vi "Find_Beam_Max_Pos.vi"(3 "Mode":T5, 4 "Beams to peak up":i32[](array[numeric]), 5 "Traverse line In":T2 {"Carrier_2 Q (l/min)" format="%#.2f"; "Row Duration (mins)" format="%#.1f"; "Row No" min=0; "Trace Gas Concentration (%)" min=0.0 format="%#_4f"; "Carrier_1 Q (l/min)" format="%#.4f"; "Start X" format="%#.2f"; "Start Y" format="%#.2f"; "Start Z" format="%#.2f"; "End X" format="%#.2f"; "End Y" format="%#.2f"; "End Z" format="%#.2f"; "Tunnel Speed" format="%#.2f"; "Averaging time (mins)" min=0.0 format="%#.2f"}) -> (0 "Error Message":string, 1 "Status":T1, 2 "Traverse line Out":T2 {"Carrier_2 Q (l/min)" format="%#.2f"; "Row Duration (mins)" format="%#.1f"; "Row No" min=0; "Trace Gas Concentration (%)" min=0.0 format="%#_4f"; "Carrier_1 Q (l/min)" format="%#.4f"; "Start X" format="%#.2f"; "Start Y" format="%#.2f"; "Start Z" format="%#.2f"; "End X" format="%#.2f"; "End Y" format="%#.2f"; "End Z" format="%#.2f"; "Tunnel Speed" format="%#.2f"; "Averaging time (mins)" min=0.0 format="%#.2f"})   [LabVIEW 2020]
uses:
  Gen Trav/Traverse_cluster.ctl
  Gen Trav/Spacing.ctl
  Controls/Multi_run_mode.ctl
  Controls/User_Specific_mode.ctl
  Gen Trav/Multi_Run_Status.ctl
  ADAM Client/Sub VIs/ADAM Controls/Remember_value_mode.ctl
  Gen Trav/Trav_mode.ctl
  Controls/Tunnel_Coordinates.ctl
  Globals/Meas_global.vi
  Globals/Preference_global.vi
  Utilities/Email_transfer_global.vi
panel:
  out "Beam Number":i32
  out "Traverse Name":string
  out "Picture Log":path
  out "First Call":bool
  out "Beam Data":dbl[][](array[numeric]) format="%.2f"
  in  "Index":i32
  # "X                Y                 Z        Datum Power"
  # "Green Unshifted\nGreen Shifted\nBlue Unshifted\nBlue Shifted"
  # "X           Y          Z"
  # "Start"
  # "End"
  # "X           Y          Z"
  # "Start"
  # "End"
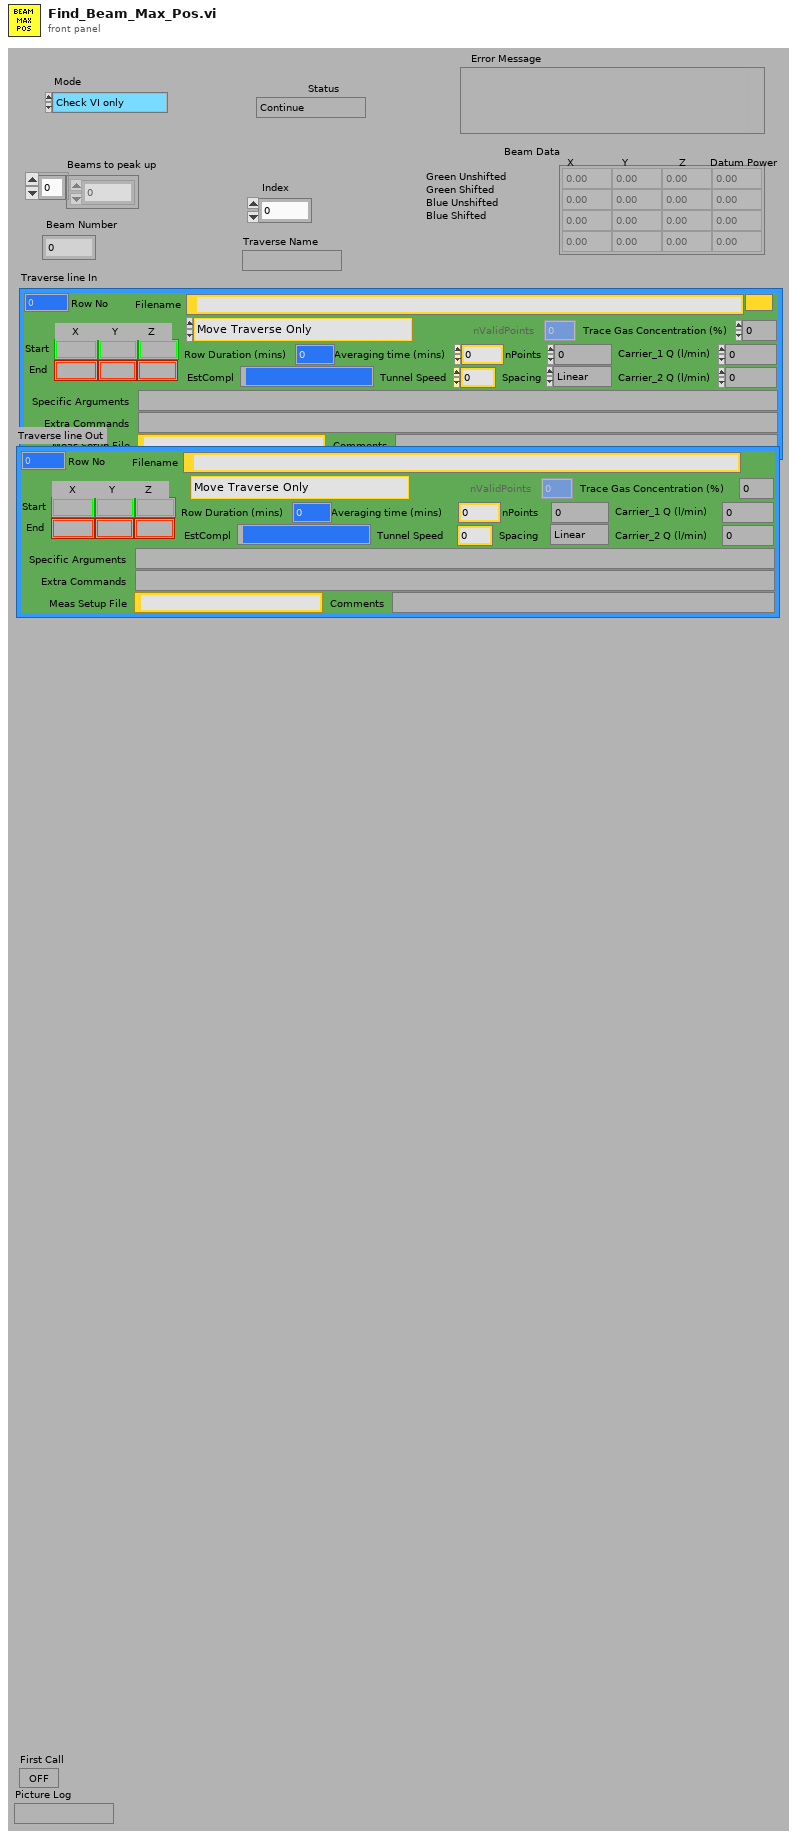
[diagram p1: front panel]
types:
  T1 = typedef "Multi_Run_Status.ctl" = enum16{"Continue", "Continue with Error", "Jump to Next Point", "Jump to Next Row", "Jump To Fall Back", "Terminate Run"}
  T2 = typedef "Traverse_cluster.ctl" = cluster{"Start X":sgl, "Start Y":sgl, "Start Z":sgl, "End X":sgl, "End Y":sgl, "End Z":sgl, "nPoints":i32, "Spacing":T3, "Filename":path, "Tunnel Speed":dbl, "Averaging time (mins)":dbl, "Extra Commands":string, "Carrier_1 Q (l/min)":dbl, "Carrier_2 Q (l/min)":dbl, "Trace Gas Concentration (%)":dbl, "Specific Arguments":string, "Comments":string, "Row No":i32, "Row Type Selector":T4, "EstCompl":string, "Row Duration (mins)":dbl, "nValidPoints":i32, "Meas Setup File":string}
  T3 = typedef "Spacing.ctl" = enum16{"Linear", "Log", "Gauss", "Specified", "N/A"}
  T4 = typedef "Multi_run_mode.ctl" = enum16{"Move Traverse Only", "Set Tunnel Speed Only", "Set Source Only", "Set Measurement Conditions", "Single Measurement", "Vertical Profile", "Lateral Profile", "Longitudinal Profile", "Multi-Axis Profile", "Explore Volume", "Auto Calibrate", "Meas Fast FID Bkgnd", "Check Beam Power", "Scanning Valve Measurement", "Run VI Named:", "Set ADAM Ch", "Wait (minutes)", "Send Message", "Synchronize With:", "Fall Back to this Row", "Turn Off Row Repeating", "Traverse 3D Volume", "Blank Row", "Jump to Fall Back Row"}
  T5 = typedef "User_Specific_mode.ctl" = enum16{"Check VI only", "Run VI"}
  T6 = typedef "Fixed Axis.ctl" = enum16{"X Axis Fixed", "Y Axis Fixed", "Z Axis Fixed"}
  T7 = cluster{"Position":dbl[], "Traverse Name":string}[][]
  T8 = typedef "Remember_value_mode.ctl" = enum16{"Read only", "Read and Write"}
  T9 = typedef "Tunnel_Coordinates.ctl" = enum16{"Work in Tunnel Coordinates", "Work in Model Coordinates"}
  T10 = typedef "Trav_mode.ctl" = enum16{"Move traverse", "Read traverse position", "Teach Position"}
  T11 = cluster{"second":i32, "minute":i32, "hour":i32, "day of month":i32, "month":i32, "year":i32, "day of week":i32, "day of year":i32, "is DST":i32}
  T12 = cluster{"Position":dbl[], "Traverse Name":string}[]
  T13 = cluster{"Position":dbl[], "Traverse Name":string}
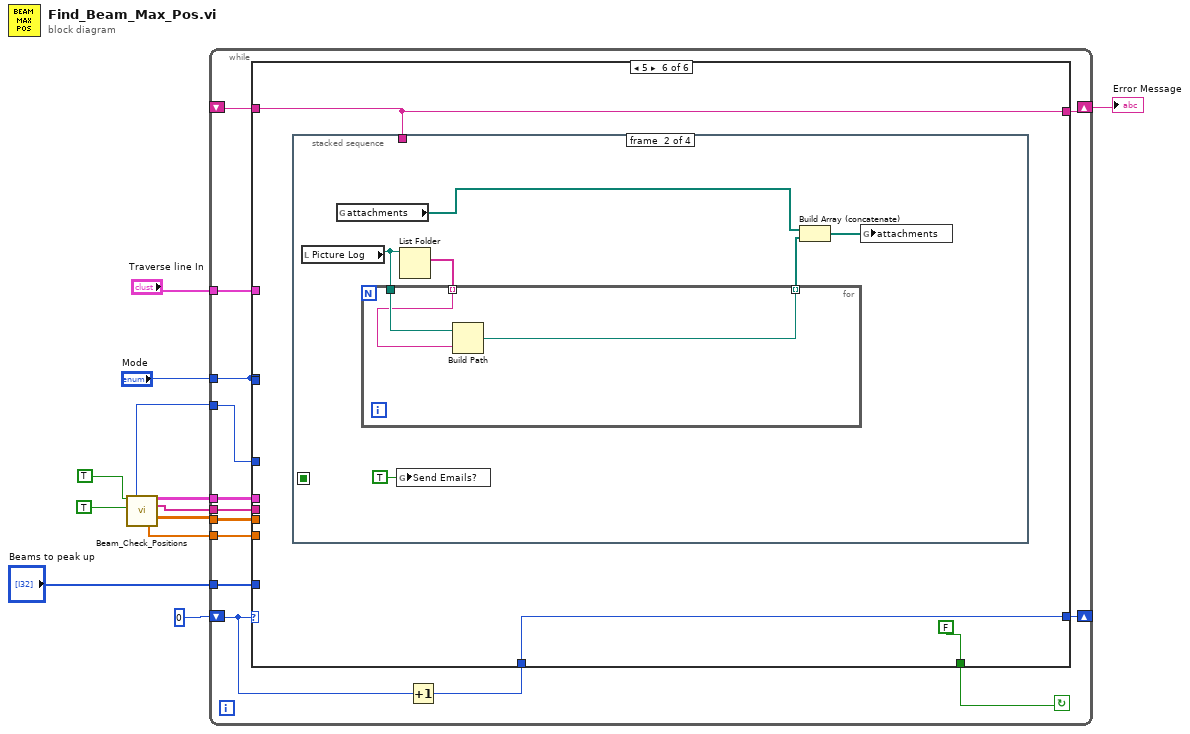
[diagram p0: block diagram]
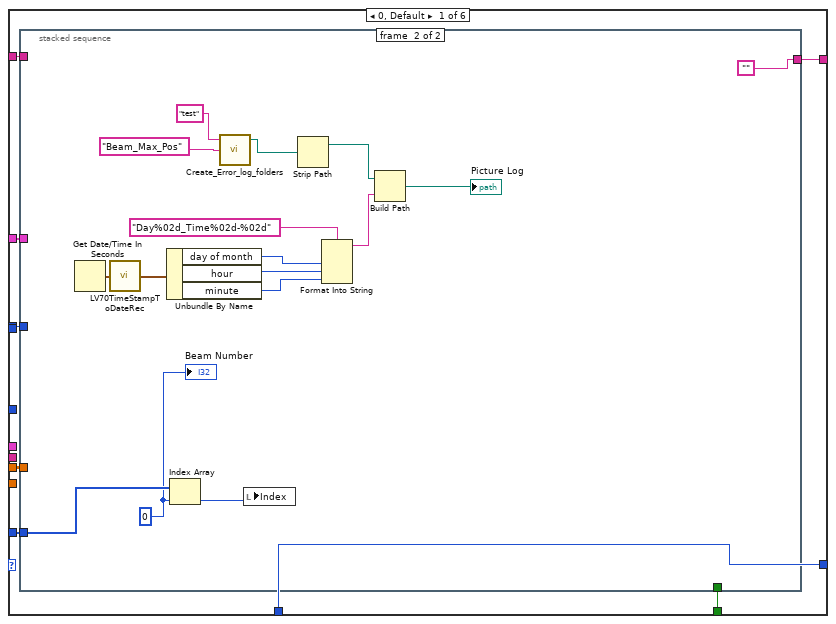
[diagram p2: hidden frame]
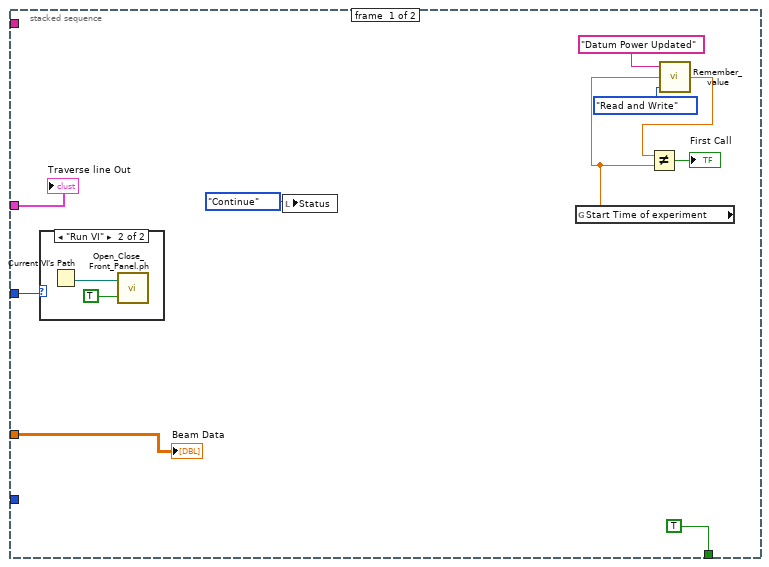
[diagram p3: hidden frame]
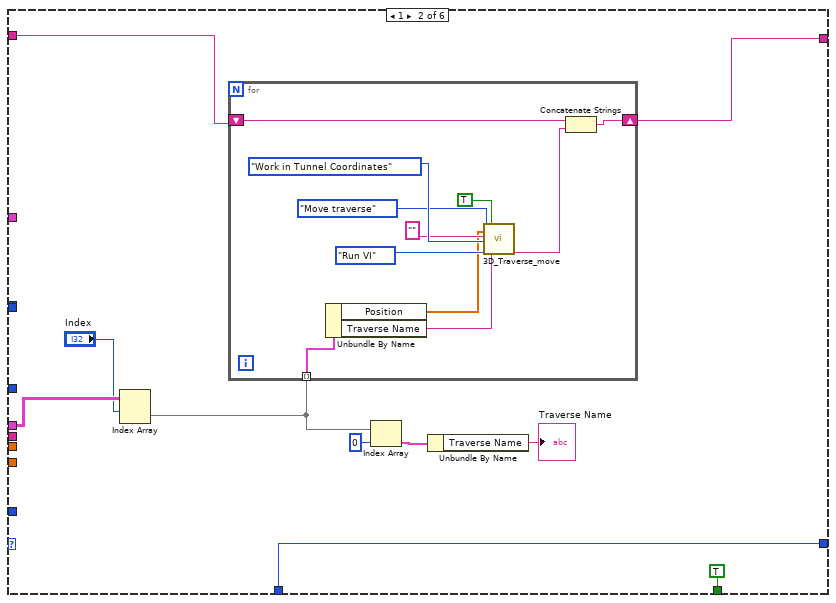
[diagram p5: hidden frame]
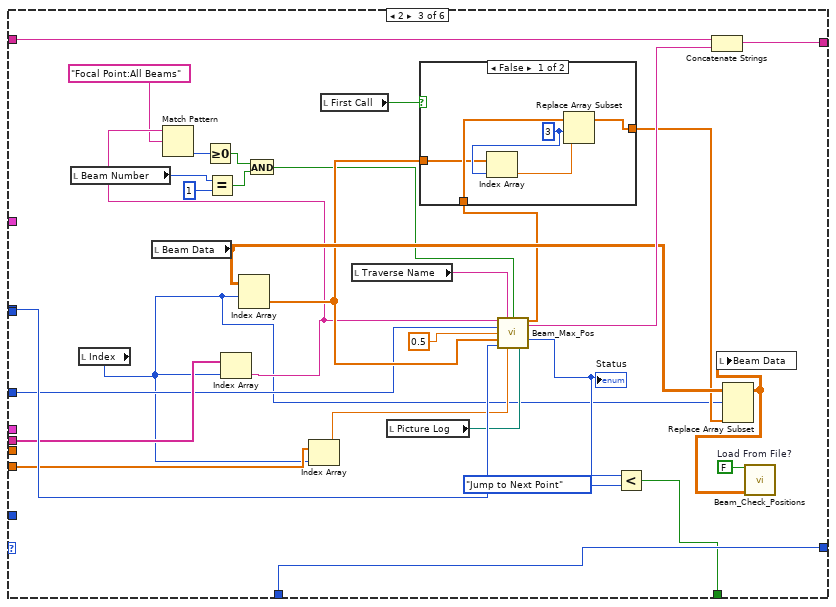
[diagram p6: hidden frame]
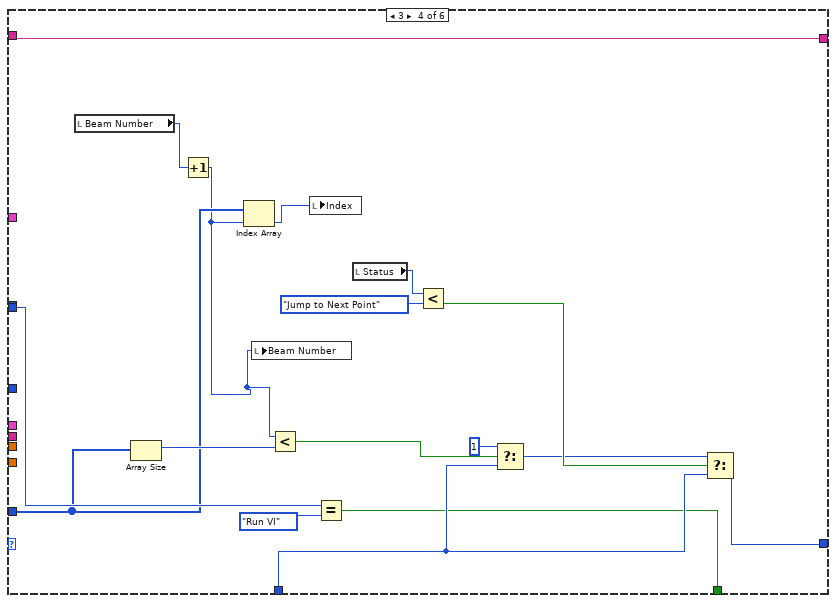
[diagram p8: hidden frame]
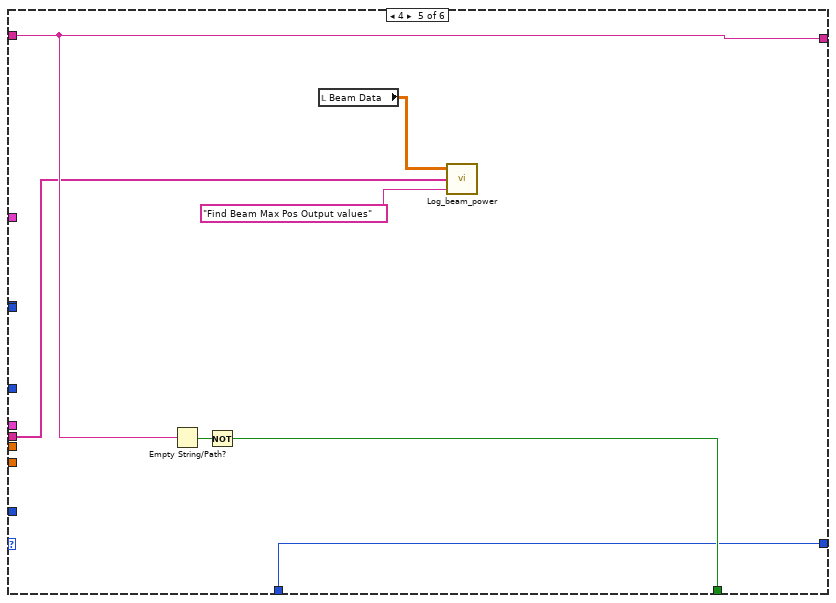
[diagram p9: hidden frame]
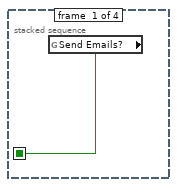
[diagram p10: hidden frame]
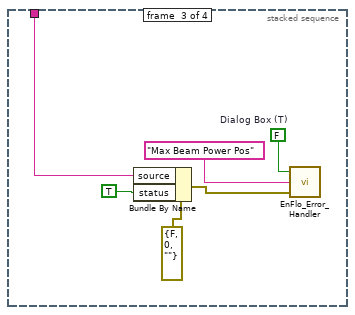
[diagram p11: hidden frame]
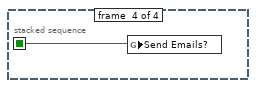
[diagram p12: hidden frame]
diagram:
  n1 = call "Beam_Check_Positions.vi"("Load From File?"=TRUE, "Give Focal Point Info (F)"=TRUE) -> ("Fixed Axis"=w8:T6, "Beam Info"=w5:T7, "Beam Names"=w2:string[], "Primary Beam Positions"=w4:dbl[][], "Wavelength (nm)"=w3:dbl[])  [unwired: 5 in, 4 out]
  n2 = while {
    shift-left: _ -> [w19]
    shift-right: [w20] -> w7
    tunnel: "Traverse line In" -> [w25]
    tunnel: "Mode" -> [w21]
    shift-left: 0 -> [w26]
    shift-right: [w22] -> _
    tunnel: w2 -> [w18]
    tunnel: w3 -> [w17]
    tunnel: w4 -> [w16]
    tunnel: w5 -> [w15]
    tunnel: w8 -> [w14]
    tunnel: "Beams to peak up" -> [w13]
    stop <- w24 continue-if-true
    n3 = Increment(x=w26) -> (x+1=w23:i32)
    n4 = case shown="5" w26 {
      tunnel: w25 -> [w31 _ _ _ _ _]
      tunnel: w21 -> [w33 _ w113 _ _ _]
      tunnel: [w32 TRUE w107 w129 w140 FALSE] -> w24
      tunnel: w23 -> [w34 w64 w114 w133 w139 w147]
      tunnel: [w34 w64 w114 w132 w139 w147] -> w22
      tunnel: w21 -> [_ _ _ w130 _ _]
      tunnel: [w30 w65 w110 w127 w142 w145] -> w20
      tunnel: w19 -> [w28 w66 w112 w127 w142 w145]
      tunnel: w18 -> [_ _ w98 _ w138 _]
      tunnel: w17 -> [_ _ w97 _ _ _]
      tunnel: w16 -> [w29 _ _ _ _ _]
      tunnel: w15 -> [_ w68 _ _ _ _]
      tunnel: w14 -> [_ _ w94 _ _ _]
      tunnel: w13 -> [w27 _ _ w123 _ _]
      frame 0, Default {
        n5 = stacked-sequence {
          tunnel: w33 -> [w43 _]
          tunnel: [TRUE _] -> w32
          tunnel: w31 -> [w42 _]
          tunnel: [_ ""] -> w30
          tunnel: w29 -> [w36 _]
          tunnel: w28 -> [_ _]
          tunnel: w27 -> [_ w49]
          frame #0 {
            n6 = case shown="\"Run VI\"" w43 {
              frame "Check VI only" {
              }
              frame "Run VI" {
                n7 = Current VI's Path() -> (path=w45:path)
                n8 = call "Open_Close_Front_Panel.ph.vi"("openWindow (T)"=TRUE ("Front Panel Window:Open"), "VI path"=w45) -> ()  [unwired: 2 out]
              }
            }
            n9 = local write "Status"(Multi_Run_Status."Continue" ("Status")) -> ()
            n10 = global read "Meas_global.vi" "Start Time of experiment"() -> (w38:dbl)
            n11 = call "Remember_value.vi"("Mode"=Remember_value_mode."Read and Write", "Input Value"=w38, "Ch name"="Datum Power Updated") -> ("Output Value"=w39:dbl)
            n12 = Not Equal?(x=w39, y=w38) -> (x != y?=→"First Call":bool)
            "Beam Data" <- w36
            "Traverse line Out" <- w42
          }
          frame #1 {
            w47 = 0 ("Index")
            n13 = Get Date/Time In Seconds() -> (seconds since 1Jan1904=w52:timestamp)
            n14 = call <vilib>:"LV70TimeStampToDateRec.vi"("time stamp"=w52) -> ("date time rec"=w60:T11)
            n15 = Unbundle By Name(w60) -> ("day of month"=w57:i32, "hour"=w58:i32, "minute"=w59:i32)
            n16 = Index Array(array=w49, index=w47) -> (element=w48:i32)
            n17 = call "Create_Error_log_folders.vi"("Log Filename"="test", "Log Folder"="Beam_Max_Pos" ("name or relative path")) -> ("Local Log File"=w51:path)  [unwired: 4 in, 1 out]
            n18 = local write "Index"(w48) -> ()
            n19 = Strip Path(path=w51) -> (stripped path=w61:path)  [unwired: 1 out]
            n20 = Format Into String(format string="Day%02d_Time%02d-%02d", w57, w58, w59) -> (resulting string=w62:string)  [unwired: 2 in, 1 out]
            n21 = Build Path(base path=w61, name or relative path=w62) -> (appended path=→"Picture Log":path)
            "Beam Number" <- w47
          }
        }
      }
      frame 1 {
        n22 = Index Array(array=w68, index (row)="Index") -> (element=w72:T12)  [unwired: 1 in]
        n23 = for {
          tunnel: w72 -> [w78] mode=indexing
          shift-right: [w75] -> w65
          shift-left: w66 -> [w74]
          n24 = Unbundle By Name(w78) -> ("Position"=w77:dbl[], "Traverse Name"=w76:string)
          n25 = call "3D_Traverse_move.vi"("Mode"=Trav_mode."Move traverse", "Position"=w77, "Extra command String"="", "Work in Tunnel Coordinates"=Tunnel_Coordinates."Work in Tunnel Coordinates", "Simulate/Run"=User_Specific_mode."Run VI", "Route Checking?"=TRUE, "Traverse name"=w76) -> ("Error String"=w73:string)  [unwired: 9 in, 3 out]
          n26 = Concatenate Strings(w74, w73) -> (w75:string)
        }
        n27 = Index Array(array=w72, index=0) -> (element=w71:T13)
        n28 = Unbundle By Name(w71) -> ("Traverse Name"=→"Traverse Name":string)
      }
      frame 2 {
        w99 = FALSE  # Load From File?
        n29 = local read "Beam Number"() -> (w87:i32)
        n30 = local read "Index"() -> (w89:i32)
        n31 = local read "Beam Data"() -> (w105:dbl[][])
        n32 = Equal?(x=w87, y=1) -> (x = y?=w85:bool)
        n33 = Index Array(array=w98, index=w89) -> (element=w92:string)
        n34 = Match Pattern(string=w92, regular expression="Focal Point:All Beams") -> (offset past match=w90:i32)  [unwired: 1 in, 3 out]
        n35 = Greater Or Equal To 0?(x=w90) -> (x >= 0?=w86:bool)
        n36 = Index Array(array=w105, index (row)=w89) -> (element=w100:dbl[])  [unwired: 1 in]
        n37 = And(x=w86, y=w85) -> (x .and. y?=w84:bool)
        n38 = Index Array(array=w97, index=w89) -> (element=w96:dbl)
        n39 = local read "First Call"() -> (w104:bool)
        n40 = local read "Traverse Name"() -> (w95:string)
        n41 = local read "Picture Log"() -> (w106:path)
        n42 = call "Beam_Max_Pos.vi"("Beam Name"=w92, "Traverse Name"=w95, "Fixed Axis only?"=w84, "Fixed Axis"=w94, "Search Step (mm)"=0.5, "Starting Position"=w100, "Mode"=w113, "Wavelength  nm"=w96, "Picture Log"=w106) -> ("Message"=w111:string, "Beam maxima"=w102:dbl[], "Status"=w108:T1)  [unwired: 3 in, 1 out]
        "Status" <- w108
        n43 = case shown="False" w104 {
          tunnel: [w118 w120] -> w103
          tunnel: w102 -> [w119 w120]
          tunnel: w100 -> [w116 _]
          frame False {
            w117 = 3 ("index")
            n44 = Index Array(array=w116, index=w117) -> (element=w115:dbl)
            n45 = Replace Array Subset(array=w119, new element=w115, index=w117) -> (w118:dbl[])
          }
          frame True {
          }
        }
        n46 = Less?(x=w108, y=Multi_Run_Status."Jump to Next Point" ("Status")) -> (x < y?=w107:bool)
        n47 = Concatenate Strings(w112, w111) -> (w110:string)
        n48 = Replace Array Subset(array=w105, new element=w103, index (row)=w89) -> (w101:dbl[][])  [unwired: 1 in]
        n49 = local write "Beam Data"(w101) -> ()
        n50 = call "Beam_Check_Positions.vi"("Load From File?"=w99, "Primary Positions In"=w101) -> ()  [unwired: 5 in, 9 out]
      }
      frame 3 {
        n51 = local read "Beam Number"() -> (w124:i32)
        n52 = Array Size(array=w123) -> (size(s)=w126:i32)
        n53 = Increment(x=w124) -> (x+1=w122:i32)
        n54 = Index Array(array=w123, index=w122) -> (element=w121:i32)
        n55 = local write "Beam Number"(w122) -> ()
        n56 = Less?(x=w122, y=w126) -> (x < y?=w125:bool)
        n57 = local write "Index"(w121) -> ()
        n58 = Equal?(x=w130, y=User_Specific_mode."Run VI" ("Mode")) -> (x = y?=w129:bool)
        n59 = local read "Status"() -> (w137:T1)
        n60 = Less?(x=w137, y=Multi_Run_Status."Jump to Next Point" ("Status")) -> (x < y?=w135:bool)
        n61 = Select(t=1, s=w125, f=w133) -> (s? t:f=w134:i32)
        n62 = Select(t=w134, s=w135, f=w133) -> (s? t:f=w132:i32)
      }
      frame 4 {
        n63 = Empty String/Path?(string/path=w142) -> (empty?=w141:bool)
        n64 = Not(x=w141) -> (.not. x?=w140:bool)
        n65 = local read "Beam Data"() -> (w144:dbl[][])
        n66 = call "Log_beam_power.vi"("Message"="Find Beam Max Pos Output values", "Beam Names"=w138, "Beam Data"=w144) -> ()  [unwired: 3 out]
      }
      frame 5 {
        n67 = stacked-sequence {
          seq-local: [w148 _ _ _] -> [_ _ _ w164]
          tunnel: w145 -> [_ _ w158 _]
          frame #0 {
            n68 = global read "Preference_global.vi" "Send Emails?"() -> (w148:bool)
          }
          frame #1 {
            n69 = local read "Picture Log"() -> (w151:path)
            n70 = global read "Email_transfer_global.vi" "attachments"() -> (w152:path[])
            n71 = global write "Preference_global.vi" "Send Emails?"(TRUE ("Send Emails?")) -> ()
            n72 = List Folder(path=w151) -> (filenames=w150:string[])  [unwired: 1 in, 5 out]
            n73 = for {
              tunnel: [w155] -> w154 mode=indexing
              tunnel: w151 -> [w157]
              tunnel: w150 -> [w156] mode=indexing
              n74 = Build Path(base path=w157, name or relative path=w156) -> (appended path=w155:path)
            }
            n75 = Build Array (concatenate)(w152, w154) -> (w153:path[])
            n76 = global write "Email_transfer_global.vi" "attachments"(w153) -> ()
          }
          frame #2 {
            w162 = FALSE  # Dialog Box (T)
            n77 = Bundle By Name(cluster=errorcluster {"status"=FALSE, "code"=0, "source"=""} ("error in (no error)"), "source"=w158, "status"=TRUE ("Bundle Element")) -> (w160:errorcluster)
            n78 = call "EnFlo_Error_Handler.vi"("error in (no error)"=w160, "Error Type"="Max Beam Power Pos", "Dialog Box (F)"=w162) -> ()  [unwired: 3 out]
          }
          frame #3 {
            n79 = global write "Preference_global.vi" "Send Emails?"(w164) -> ()
          }
        }
      }
    }
  }
  "Error Message" <- w7
